vi "Pause.vi"(8 "error in (no error)":errorcluster, 11 "VICI Settings In":T1 {"Pump Number" min=0.0 max=20.0 step=1.0}) -> (0 "error out":errorcluster, 3 "VICI Settings Out":T1 {"Pump Number" min=0.0 max=20.0 step=1.0})   [LabVIEW 2018, in "VICI M50.lvlib"]
uses:
  VICI M50.lvlib
  Settings Cluster.ctl
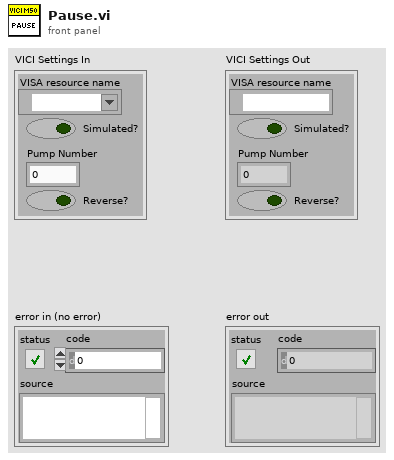
[diagram p1: front panel]
types:
  T1 = typedef "Settings Cluster.ctl" = cluster{"VISA resource name":refnum<visa-resource-name>, "Simulated?":bool, "Pump Number":dbl, "Reverse?":bool}
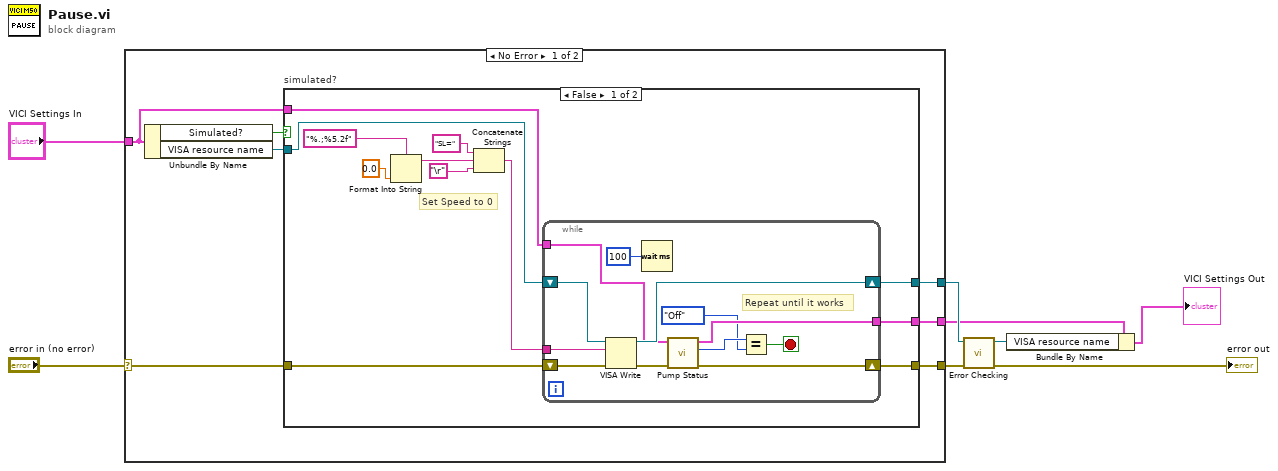
[diagram p0: block diagram]
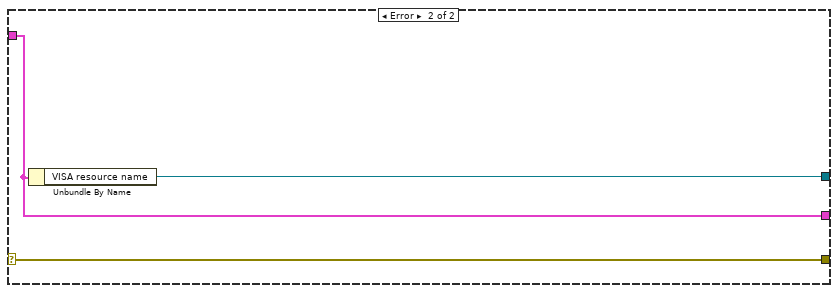
[diagram p3: hidden frame]
diagram:
  n1 = case shown="No Error" "error in (no error)" {
    selector: "error in (no error)" -> [w15 w45]
    tunnel: [w11 w44] -> w2
    tunnel: "VICI Settings In" -> [w12 w44]
    tunnel: [w14 w43] -> w6
    tunnel: [w13 w45] -> w5
    frame No Error {
      n2 = Unbundle By Name(w12) -> ("Simulated?"=w9:bool, "VISA resource name"=w10:refnum<visa-resource-name>)
      n3 = case "simulated?" shown="False" w9 {
        tunnel: [w25 w42] -> w14
        tunnel: w10 -> [w27 w42]
        tunnel: w15 -> [w26 w41]
        tunnel: [w24 w41] -> w13
        tunnel: w12 -> [w23 w40]
        tunnel: [w22 w40] -> w11
        frame False {
          # "Set Speed to 0"
          n4 = Format Into String(format string="%.;%5.2f", 0.0 ("input 1")) -> (resulting string=w21:string)  [unwired: 2 in, 1 out]
          n5 = Concatenate Strings("SL=" ("string"), w21, "\r") -> (w16:string)
          n6 = while {
            shift-right: [w37] -> w25
            shift-left: w27 -> [w39]
            shift-right: [w35] -> w24
            shift-left: w26 -> [w38]
            tunnel: w23 -> [w34]
            tunnel: [w33] -> w22
            tunnel: w16 -> [w28]
            stop <- w29 stop-if-true
            # "Repeat until it works"
            n7 = VISA Write(VISA resource name=w39, write buffer=w28, error in (no error)=w38) -> (VISA resource name out=w37:refnum<visa-resource-name>, error out=w36:errorcluster)  [unwired: 1 out]
            n8 = Wait (ms)(milliseconds to wait=u32 100) -> ()  [unwired: 1 out]
            n9 = call "Pump Status.vi"("error in (no error)"=w36, "VICI Settings In"=w34) -> ("error out"=w35:errorcluster, "Pump On?"=w31:enum16{"Off", "On", "Not Initialized"}, "VICI Settings Out"=w33:T1)  [unwired: 6 in, 1 out]
            n10 = Equal?(x=w31, y=enum16{"Off", "On", "Not Initialized"}."Off") -> (x = y?=w29:bool)
          }
        }
        frame True {
        }
      }
    }
    frame Error {
      n11 = Unbundle By Name(w44) -> ("VISA resource name"=w43:refnum<visa-resource-name>)
    }
  }
  n12 = call "Error Checking.vi"("error in (no error)"=w5, "VISA resource name"=w6) -> ("error out"=→"error out":errorcluster, "VISA resource name"=w3:refnum<visa-resource-name>)  [unwired: 7 in, 1 out]
  n13 = Bundle By Name(cluster=w2, "VISA resource name"=w3) -> (→"VICI Settings Out":T1)
